vi "RandomLaser20.vi"() -> ()   [LabVIEW 2014]
uses:
  State-MainLoop.ctl
  <userlib>/_OpenG.lib/array/array.llb/Delete Elements from 2D Array (DBL)__ogtk.vi
panel:
  in  "Tab Control":T1(tab)
  out "Intensity Graph":dbl[][](graph)
  in  "Average":i32=1
  in  "Integration Time":i32=100
  out "Spectrum":T2(graph)
  in  "Custom Marker Colors":u32[](array[colorbox])=[9567230, 1187327, 3465]
  in  "Buffer Graph":i32=30
  in  "index (row)":i32
  in  "Select Light Source":u16(ring)
  out "Power Meter (W)":dbl=0.009689930499999999 format="%#_4p"
  out "Power Graph":dbl[](graph)
  in  "StepperMotor":bool
  out "Steps Chart":dbl(graph)
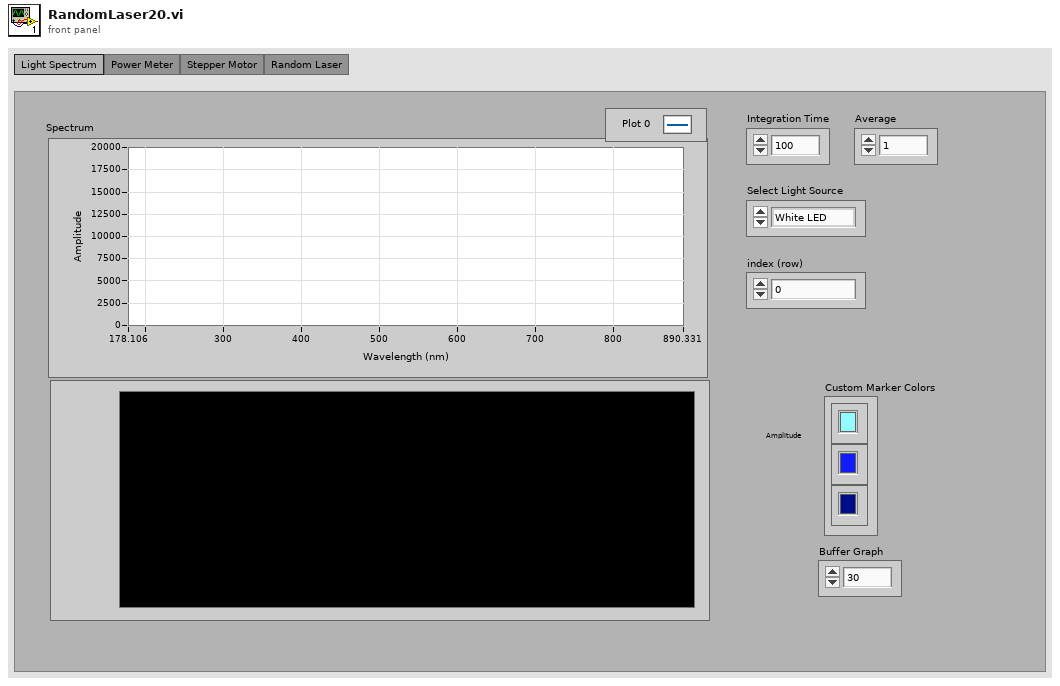
[diagram p1: front panel]
types:
  T1 = enum32{"Light Spectrum", "Power Meter", "Stepper Motor", "Random Laser"}
  T2 = cluster{"WL Values":dbl[], "Spectrum Values":dbl[]}
  T3 = typedef "State-MainLoop.ctl" = enum16{"Initialize", "Wait for Event", "Spectrum Graph", "Power Meter", "Stepper Motor", "Random Laser"}
  T4 = enum32{"Page Enabled", "Page Disabled", "Page Disabled & Grayed"}
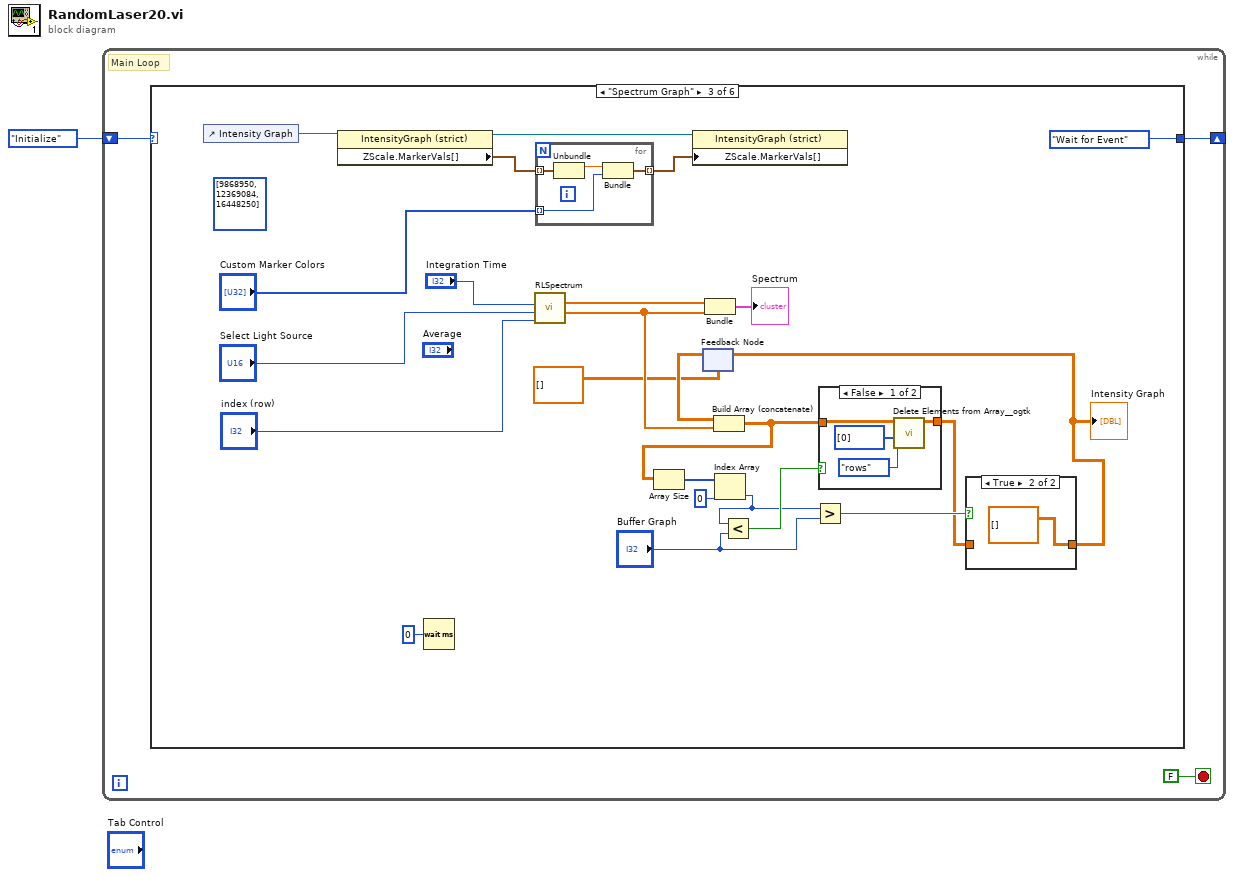
[diagram p0: block diagram]
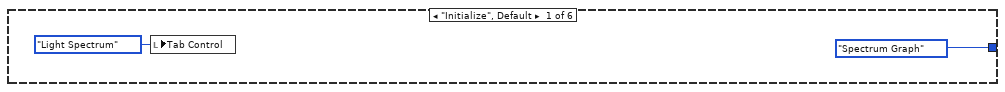
[diagram p2: hidden frame]
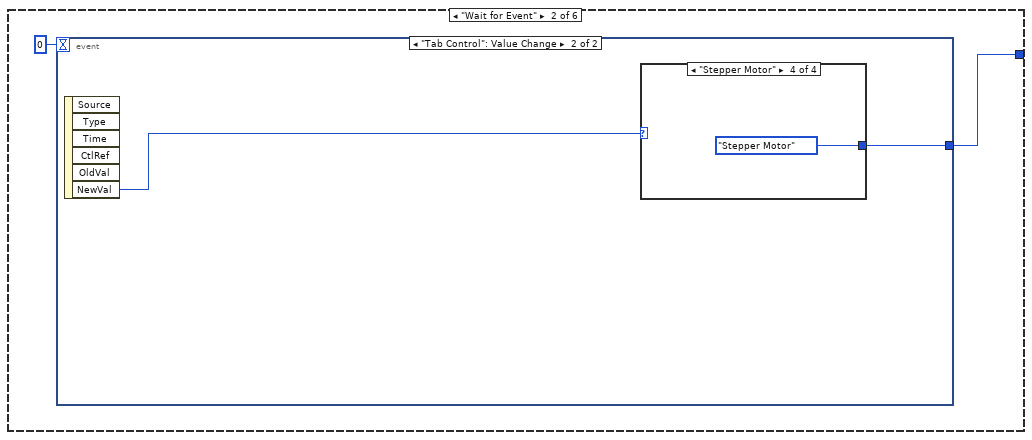
[diagram p3: hidden frame]
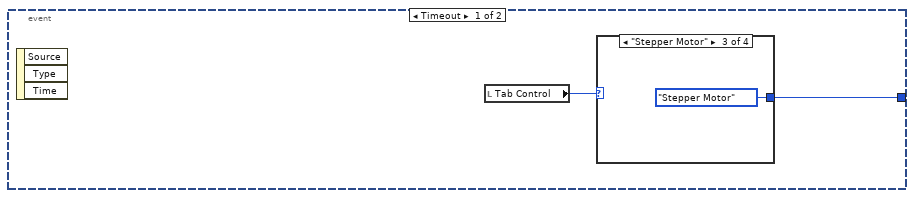
[diagram p4: hidden frame]
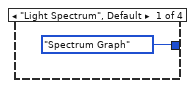
[diagram p5: hidden frame]
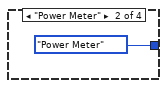
[diagram p6: hidden frame]
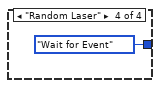
[diagram p7: hidden frame]
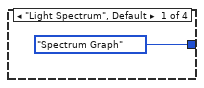
[diagram p8: hidden frame]
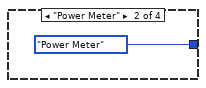
[diagram p9: hidden frame]
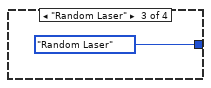
[diagram p10: hidden frame]
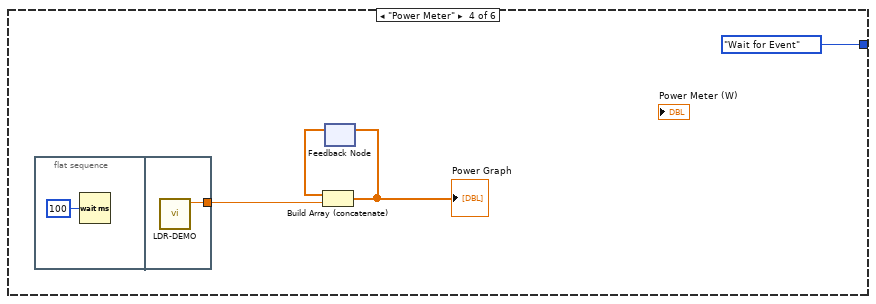
[diagram p13: hidden frame]
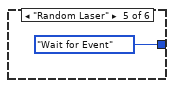
[diagram p14: hidden frame]
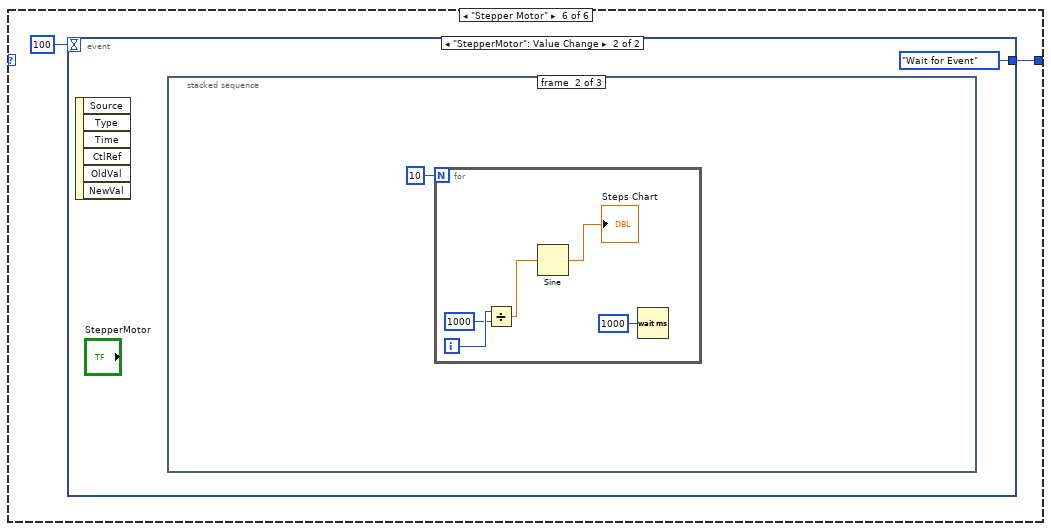
[diagram p15: hidden frame]
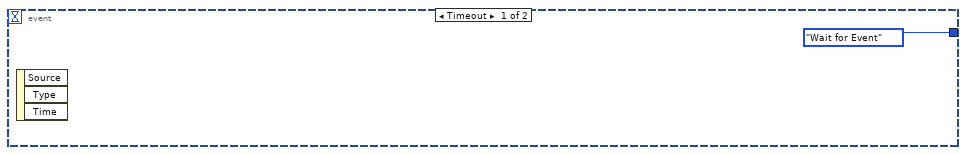
[diagram p16: hidden frame]
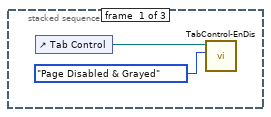
[diagram p17: hidden frame]
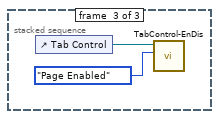
[diagram p18: hidden frame]
diagram:
  n1 = while {
    shift-right: [w2] -> _
    shift-left: State-MainLoop."Initialize" -> [w3]
    stop <- FALSE stop-if-true
    # "Main Loop"
    n2 = case shown="\"Spectrum Graph\"" w3 {
      tunnel: [State-MainLoop."Spectrum Graph" w8 State-MainLoop."Wait for Event" State-MainLoop."Wait for Event" State-MainLoop."Wait for Event" w63] -> w2
      frame "Initialize", Default {
        n3 = local write "Tab Control"(T1."Light Spectrum" ("Tab Control")) -> ()
      }
      frame "Wait for Event" {
        n4 = event shown="[1] \"Tab Control\": Value Change" {
          selector: _ -> [_ _]
          dyn-events: _ -> [_ _]
          timeout: 0 -> [_ _]
          tunnel: [w10 w15] -> w8
          event Timeout {
            n5 = event-data() -> ()  [unwired: 1 in, 3 out]
            n6 = local read "Tab Control"() -> (w9:T1)
            n7 = case shown="\"Stepper Motor\"" w9 {
              tunnel: [State-MainLoop."Spectrum Graph" State-MainLoop."Power Meter" State-MainLoop."Stepper Motor" State-MainLoop."Wait for Event"] -> w10
              frame "Light Spectrum", Default {
              }
              frame "Power Meter" {
              }
              frame "Stepper Motor" {
              }
              frame "Random Laser" {
              }
            }
          }
          event "Tab Control": Value Change {
            n8 = event-data() -> ("NewVal"=w16:T1)  [unwired: 1 in, 5 out]
            n9 = case shown="\"Stepper Motor\"" w16 {
              tunnel: [State-MainLoop."Spectrum Graph" State-MainLoop."Power Meter" State-MainLoop."Random Laser" State-MainLoop."Stepper Motor"] -> w15
              frame "Light Spectrum", Default {
              }
              frame "Power Meter" {
              }
              frame "Random Laser" {
              }
              frame "Stepper Motor" {
              }
            }
          }
        }
      }
      frame "Spectrum Graph" {
        (unwired) u32[] [9868950, 12369084, 16448250] ("Custom Marker Colors")
        n10 = control-ref of="Intensity Graph"() -> (w34:refnum<vi>)
        n11 = property on="Property Node" class="IntensityGraph (strict)"(reference=w34) -> (reference out=w32:refnum<vi>, "ZScale.MarkerVals[]"=w41:cluster{dbl, u32}[])  [unwired: 1 in, 1 out]
        n12 = Wait (ms)(milliseconds to wait=u32 0) -> ()  [unwired: 1 out]
        n13 = call "RLSpectrum.vi"("index (row)"="index (row)", "Select Light Source"="Select Light Source", "Integration Time (ms)"="Integration Time") -> ("Spectrum Values"=w30:dbl[], "WL Values"=w29:dbl[])  [unwired: 7 in]
        n14 = for {
          tunnel: w41 -> [w55] mode=indexing
          tunnel: "Custom Marker Colors" -> [w53] mode=indexing
          tunnel: [w52] -> w40 mode=indexing
          n15 = Unbundle(w55) -> (w54:dbl)  [unwired: 1 out]
          n16 = Bundle(w54, "Color Box"=w53) -> (w52:cluster{dbl, "Color Box":u32})  [unwired: 1 in]
        }
        n17 = property on="Property Node" class="IntensityGraph (strict)"(reference=w32, "ZScale.MarkerVals[]"=w40) -> ()  [unwired: 1 in, 2 out]
        n18 = feedback #1(dbl[][] []) -> (w42:dbl[][])
        n19 = Bundle("WL Values"=w29, "Spectrum Values"=w30) -> (→"Spectrum":T2)  [unwired: 1 in]
        n20 = Build Array (concatenate)(w42, w30) -> (w38:dbl[][])
        n21 = Array Size(array=w38) -> (size(s)=w37:i32[])
        n22 = Index Array(array=w37, index=0) -> (element=w27:i32)
        n23 = Less?(x=w27, y="Buffer Graph") -> (x < y?=w35:bool)
        n24 = Greater?(x=w27, y="Buffer Graph") -> (0:w25:bool)
        n25 = case shown="False" w35 {
          tunnel: w38 -> [w50 w51]
          tunnel: [w49 w51] -> w24
          frame False {
            n26 = call-poly <userlib>:"Delete Elements from Array__ogtk.vi"("delete (rows or columns)"=enum16{"rows", "columns"}."rows", "indices"=i32[] [0], "array"=w50) -> ("array w/ subset deleted"=w49:dbl[][])  [unwired: 7 in, 1 out]
          }
          frame True {
          }
        }
        n27 = case shown="True" w25 {
          tunnel: w24 -> [w45 _]
          tunnel: [w45 dbl[][] []] -> w23
          frame False {
          }
          frame True {
          }
        }
        "Intensity Graph" <- w23
        n28 = feedback-in #1(w23) -> ()
      }
      frame "Power Meter" {
        n29 = flat-sequence {
          tunnel: [w61] -> w57
          frame #0 {
            n30 = Wait (ms)(milliseconds to wait=u32 100) -> ()  [unwired: 1 out]
          }
          frame #1 {
            n31 = call "LDR-DEMO.vi"() -> ("Voltage"=w61:dbl)  [unwired: 10 in, 1 out]
          }
        }
        n32 = feedback #2() -> (w58:dbl[])  [unwired: 1 in]
        n33 = Build Array (concatenate)(w58, w57) -> (w56:dbl[])
        "Power Graph" <- w56
        n34 = feedback-in #2(w56) -> ()
      }
      frame "Random Laser" {
      }
      frame "Stepper Motor" {
        n35 = event shown="[1] \"StepperMotor\": Value Change" {
          selector: _ -> [_ _]
          dyn-events: _ -> [_ _]
          timeout: 100 -> [_ _]
          tunnel: [State-MainLoop."Wait for Event" State-MainLoop."Wait for Event"] -> w63
          event Timeout {
            n36 = event-data() -> ()  [unwired: 1 in, 3 out]
          }
          event "StepperMotor": Value Change {
            n37 = event-data() -> ()  [unwired: 1 in, 6 out]
            n38 = stacked-sequence {
              frame #0 {
                n39 = control-ref of="Tab Control"() -> (w67:refnum<vi>)
                n40 = call "TabControl-EnDis.vi"("Page Enabled State"=T4."Page Disabled & Grayed", "TabControl in"=w67) -> ()  [unwired: 9 in, 1 out]
              }
              frame #1 {
                n41 = for {
                  N: 10 -> [_]
                  i -> [w74]
                  n42 = Divide(x=w74, y=1000) -> (x/y=w72:dbl)
                  n43 = Sine(x=w72) -> (sin(x)=→"Steps Chart":dbl)
                  n44 = Wait (ms)(milliseconds to wait=u32 1000) -> ()  [unwired: 1 out]
                }
              }
              frame #2 {
                n45 = control-ref of="Tab Control"() -> (w75:refnum<vi>)
                n46 = call "TabControl-EnDis.vi"("Page Enabled State"=T4."Page Enabled", "TabControl in"=w75) -> ()  [unwired: 9 in, 1 out]
              }
            }
          }
        }
      }
    }
  }
